vi "Find Bracket Pairs.vi"(11 "BrainTease Script":string) -> (0 "Error":bool, 1 "Ket":u64[](array[numeric]), 2 "Bra":u64[](array[numeric]), 3 "BraKet Pairs":T1[](array[typedef]))   [LabVIEW 2019]
uses:
  BraKet Pair.ctl
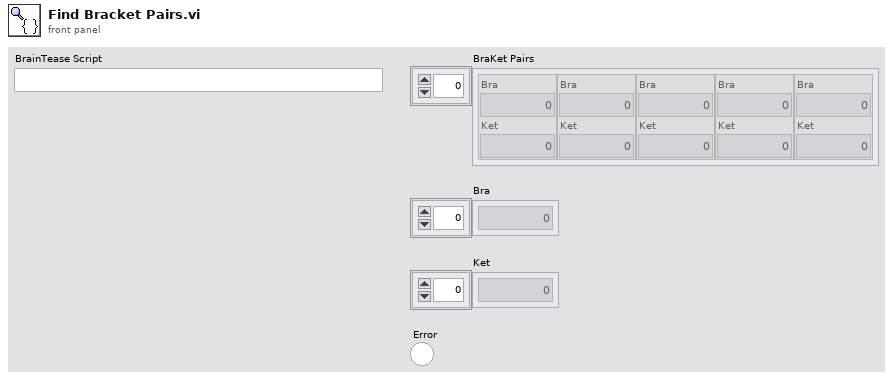
[diagram p1: front panel]
types:
  T1 = typedef "BraKet Pair.ctl" = cluster{"Bra":u64, "Ket":u64}
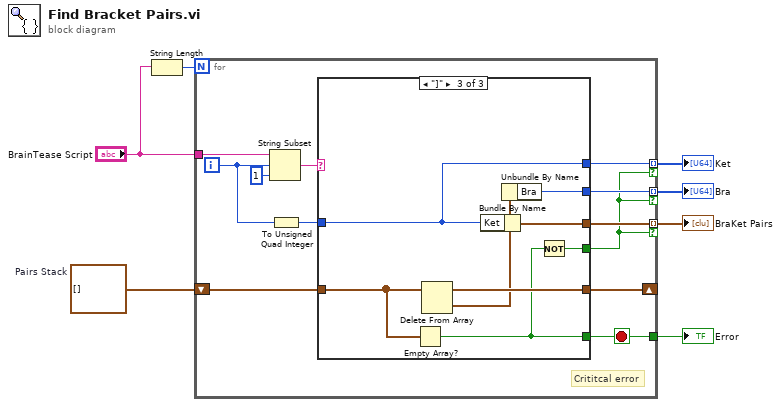
[diagram p0: block diagram]
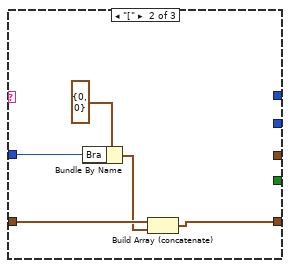
[diagram p3: hidden frame]
diagram:
  w5 = T1[] []  # Pairs Stack
  n1 = String Length(string="BrainTease Script") -> (length=w7:i32)
  n2 = for {
    N: w7 -> [_]
    tunnel: "BrainTease Script" -> [w19]
    shift-right: [w16] -> _
    shift-left: w5 -> [w15]
    tunnel: [w12] -> w3 mode=indexing if=w8
    tunnel: [w11] -> w4
    tunnel: [w10] -> w1 mode=indexing if=w8
    tunnel: [w9] -> w2 mode=indexing if=w8
    i -> [w14]
    stop <- w11 stop-if-true
    # "Crititcal error"
    n3 = String Subset(string=w19, offset (0)=w14, length (rest)=1 ("length (rest)")) -> (substring=w17:string)
    n4 = To Unsigned Quad Integer(1:w14) -> (0:w13:u64)
    n5 = case shown="\"]\"" w17 {
      tunnel: [w20 w21 w32] -> w16
      tunnel: w15 -> [w20 w25 w31]
      tunnel: w13 -> [_ w23 w28]
      tunnel: [_ _ w33] -> w12
      tunnel: [_ _ w30] -> w8
      tunnel: [_ _ w29] -> w11
      tunnel: [_ _ w28] -> w10
      tunnel: [_ _ w26] -> w9
      frame Default {
      }
      frame "[" {
        n6 = Bundle By Name(cluster=T1 {"Bra"=0, "Ket"=0}, "Bra"=w23) -> (w22:T1)
        n7 = Build Array (concatenate)(w25, w22) -> (w21:T1[])
      }
      frame "]" {
        n8 = Empty Array?(array=w31) -> (empty?=w29:bool)
        n9 = Delete From Array(array=w31) -> (deleted portion=w27:T1, array with subset deleted=w32:T1[])  [unwired: 2 in]
        n10 = Bundle By Name(cluster=w27, "Ket"=w28) -> (w33:T1)
        n11 = Unbundle By Name(w27) -> ("Bra"=w26:u64)
        n12 = Not(x=w29) -> (.not. x?=w30:bool)
      }
    }
  }
  "BraKet Pairs" <- w3
  "Error" <- w4
  "Bra" <- w2
  "Ket" <- w1
